vi "AverageLastNvalues.vi"(10 "N":i32=5, 11 "Circle time series":dbl[][](array[numeric])) -> (3 "Average of last N array elements":dbl)   [LabVIEW 2013]
doc: "Return the average pupil diameter from Circle time series. Average is over the N (default: 5) latest samples."
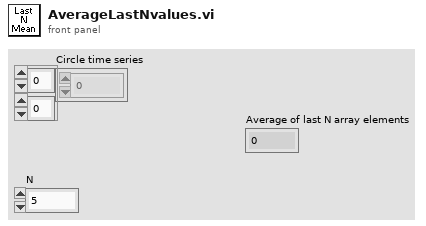
[diagram p1: front panel]
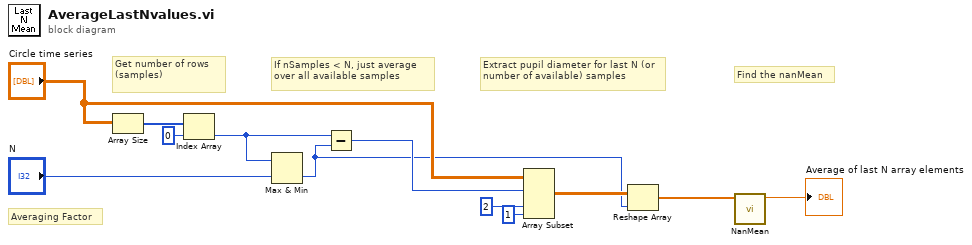
[diagram p0: block diagram]
diagram:
  # "Find the nanMean"
  # "Extract pupil diameter for last N (or number of available) samples"
  # "If nSamples < N, just average over all available samples"
  # "Averaging Factor"
  # "Get number of rows \n(samples)"
  n1 = Array Size(array="Circle time series") -> (size(s)=w4:i32[])
  n2 = Index Array(array=w4, index=0) -> (element=w9:i32)
  n3 = Max & Min(x=w9, y="N") -> (min(x,y)=w1:i32)  [unwired: 1 out]
  n4 = Subtract(x=w9, y=w1) -> (x-y=w12:i32)
  n5 = Array Subset(array="Circle time series", index (row)=w12, index (col)=2 ("disabled index (col)"), length (col)=1 ("length")) -> (w11:dbl[][])  [unwired: 1 in]
  n6 = Reshape Array(w11, w1) -> (w3:dbl[])
  n7 = call "NanMean.vi"("Array"=w3) -> ("Nanmean"=→"Average of last N array elements":dbl)  [unwired: 10 in]
